vi "Read File Path.vi"(8 "error in (no error)":errorcluster, 11 "File Writer in":refnum<class "File Writer.lvclass">) -> (0 "error out":errorcluster, 1 "Is Active?":bool, 2 "File Path":path, 3 "File Writer out":refnum<class "File Writer.lvclass">)   [LabVIEW 2020, in "File Writer.lvlib" / "File Writer.lvclass"]
doc: "Read the file path from the File Writer."
uses:
  File Writer.lvclass
  File Writer.lvclass/File Writer.ctl
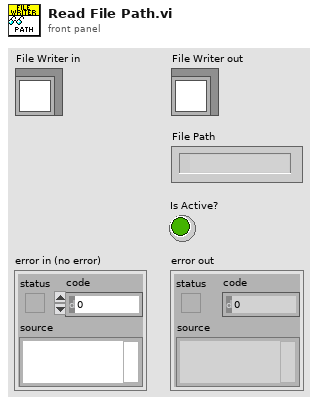
[diagram p1: front panel]
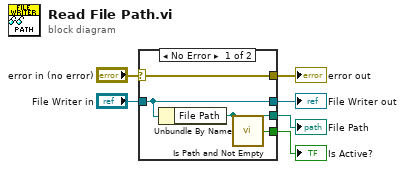
[diagram p0: block diagram]
diagram:
  n1 = case shown="No Error" "error in (no error)" {
    selector: "error in (no error)" -> [w10 w11]
    tunnel: [w10 w11] -> w5
    tunnel: [w9 w12] -> w3
    tunnel: "File Writer in" -> [w9 w12]
    tunnel: [w8 _] -> w2
    tunnel: [w7 _] -> w1
    frame No Error {
      n2 = Unbundle By Name(w9) -> ("File Path"=w8:path)
      n3 = call <vilib>:"Is Path and Not Empty.vi"("path"=w8) -> ("Is Path and Not Empty?"=w7:bool)  [unwired: 4 in]
    }
    frame Error {
    }
  }
  "error out" <- w5
  "File Writer out" <- w3
  "File Path" <- w2
  "Is Active?" <- w1
